vi "View one AI param scada restr.vi"(4 "AIParamTable":string="fa_1", 6 "OPC UA.Client refnum":T2, 7 "conninfo":T4={"host"="localhost", "port"="5432", "client_encoding"="WIN1251", "dbname"="system", "user"="postgres", "password"=""}, 8 "error in (no error)":errorcluster, 9 "AIParameters":string[](array[string]), 10 "AI_State":T3[](array[typedef]), 11 "AITable":dbl[](array[numeric]) format="%#.0f") -> (0 "error out":errorcluster)   [LabVIEW 2019]
uses:
  Ctl/AIParamColumns.ctl
  Inputs.lvlib
  <vilib>/OPCUA/controls/NodeId.ctl
  <vilib>/OPCUA/NI OPC UA Client.lvlib
  OPC/OPC addons.lvlib
  Ctl/View one AI param State.ctl
  <vilib>/Utility/miscctls.llb/LVRowAndColumnUnsignedTypeDef.ctl
  <vilib>/OPCUA/client/Multiple Write Variant.vi
  Ctl/Parameter State.ctl
  Database/ctl/Coninfo.ctl
  Database/PostgreSQL.lvlib
  <vilib>/OPCUA/controls/OPC UA Client Refnum.ctl
panel:
  in  "Tab Control":T1(tab)
  in  "input_register_min":dbl min=-32768.0 max=65535.0 step=1.0 format="%#.0f"
  in  "input_register_max":dbl min=-32768.0 max=65535.0 step=1.0 format="%#.0f"
  in  "input_pv_min":dbl format="%#.1f"
  in  "input_pv_max":dbl format="%#.1f"
  in  "instrument_gain":dbl min=-32768.0 max=65535.0 step=1.0 format="%#.0f"
  in  "instrument_offset":dbl min=-32768.0 max=65535.0 step=1.0 format="%#.0f"
  in  "sensor num":i32
  in  "instrument_min_offset":dbl min=-32768.0 max=65535.0 step=1.0 format="%#.0f"
  in  "time_const":dbl min=-32768.0 max=65535.0 step=1.0 format="%#.0f"
  in  "fcode_full":string="кгс/см2"
  out "AI_1":dbl format="%#.1f"
  in  "Param":i32(listbox) caption="Параметры"
  in  "d":dbl min=-32768.0 max=65535.0 step=1.0 format="%#.0f"
  in  "instrument_max_offset":dbl min=-32768.0 max=65535.0 step=1.0 format="%#.0f"
  out "units":string="кгс/см2"
  in  "instrument_range_max":dbl format="%#.1f"
  in  "process_range_max":dbl format="%#.1f"
  in  "process_high_acd":dbl format="%#.1f"
  in  "process_high_alr":dbl format="%#.1f"
  in  "process_low_alr":dbl format="%#.1f"
  in  "process_low_acd":dbl format="%#.1f"
  in  "process_range_min":dbl format="%#.1f"
  in  "instrument_range_min":dbl format="%#.1f"
  # "Настройка пределов"
  # "верхнийний предел датчика"
  # "верхний предел достоверных показаний"
  # "верхний аварийный предел"
  # "верхний предупредительный предел"
  # "нижний предупредительный предел"
  # "нижний аварийный предел"
  # "нижний предел достоверных показаний"
  # "нижний предел датчика"
  # "Y"
  # "значение сигнала максимум (Ymax)"
  # "значение сигнала минимум (Ymin)"
  # "X"
  # "входной регистр минимум (Xmin)"
  # "входной регистр максимум (Xmax)"
  # "Y"
  # "массштабирование"
  # "смещение"
  # "X"
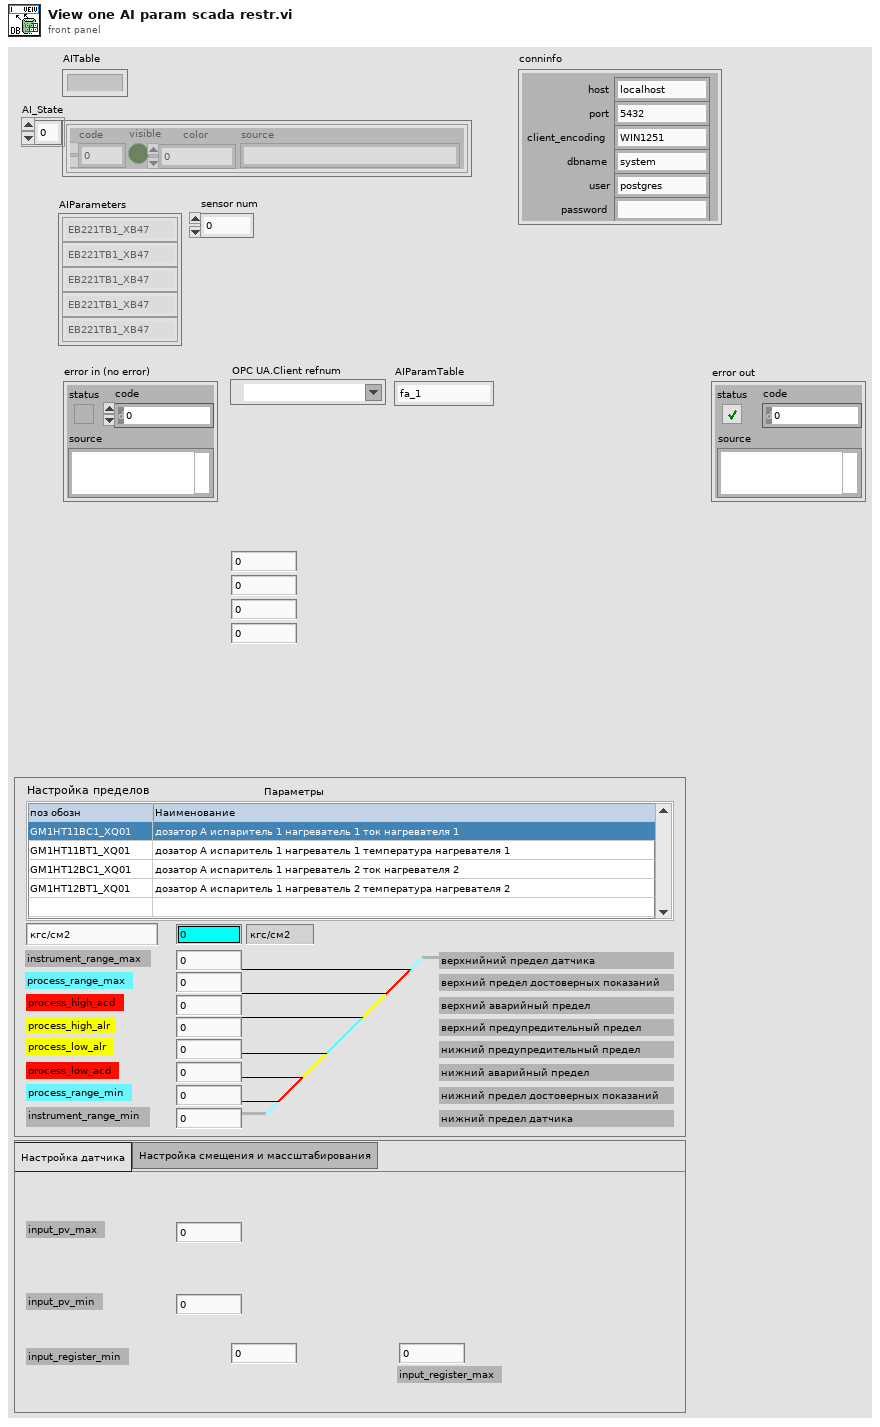
[diagram p1: front panel]
types:
  T1 = enum32{"Настройка датчика", "Настройка смещения и массштабирования"}
  T2 = typedef "OPC UA Client Refnum.ctl" = refnum<k21>
  T3 = typedef "Inputs.lvlib/Parameter State.ctl" = cluster{"code":i32, "visible":bool, "color":u32, "source":string}
  T4 = typedef "PostgreSQL.lvlib/Coninfo.ctl" = cluster{"host":string, "port":string, "client_encoding":string, "dbname":string, "user":string, "password":string}
  T5 = typedef "Inputs.lvlib/View one AI param State.ctl" = enum16{"init", "change sensor", "wait changes", "write parameters"}
  T6 = typedef "LVRowAndColumnUnsignedTypeDef.ctl" = cluster{"Row":u32, "Column":u32}
  T7 = typedef "NodeId.ctl" = string
  T8 = typedef "Inputs.lvlib/AIParamColumns.ctl" = enum16{"instrument_gain", "instrument_offset", "time_const", "instrument_min_offset", "instrument_range_min", "process_range_min", "process_low_acd", "process_low_alr", "process_high_alr", "process_high_acd", "process_range_max", "instrument_range_max", "instrument_max_offset", "d", "input_register_min", "input_register_max", "input_pv_min", "input_pv_max", "module_fcode_full", "control_channel_num", "ip_adress", "fcode", "fcodef", "fcode_full", "fname", "process_units"}
  T9 = typedef "Write Variant Request.ctl" = cluster{"node ID":T7, "value":variant, "timestamp (current time)":timestamp, "node status":T10}
  T10 = typedef "Write Status.ctl" = u32
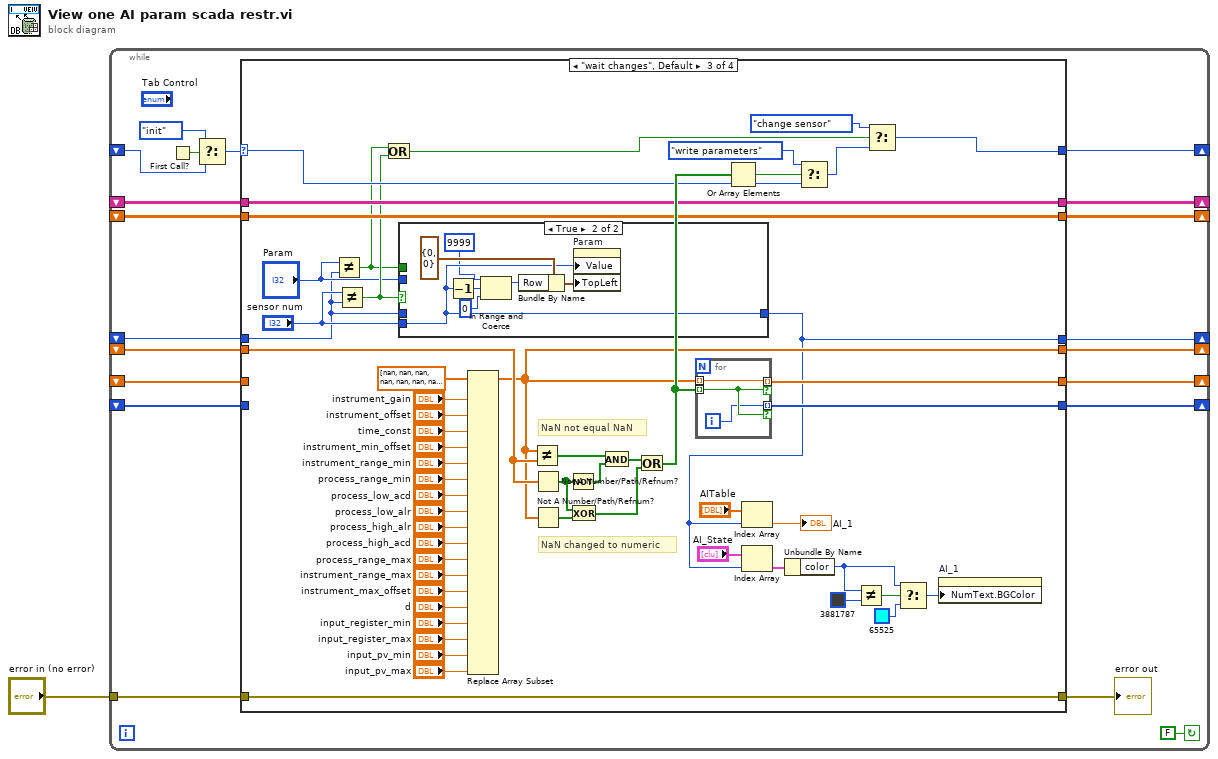
[diagram p0: block diagram]
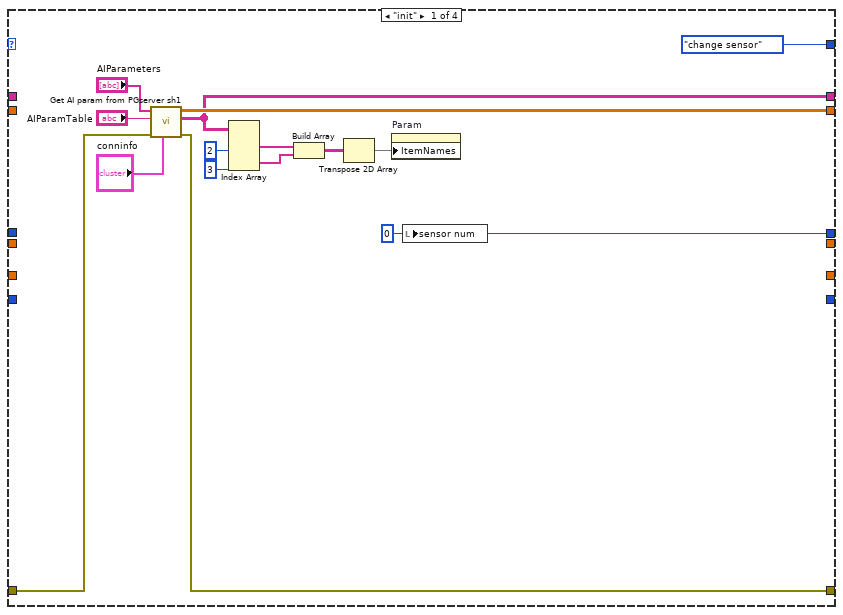
[diagram p2: hidden frame]
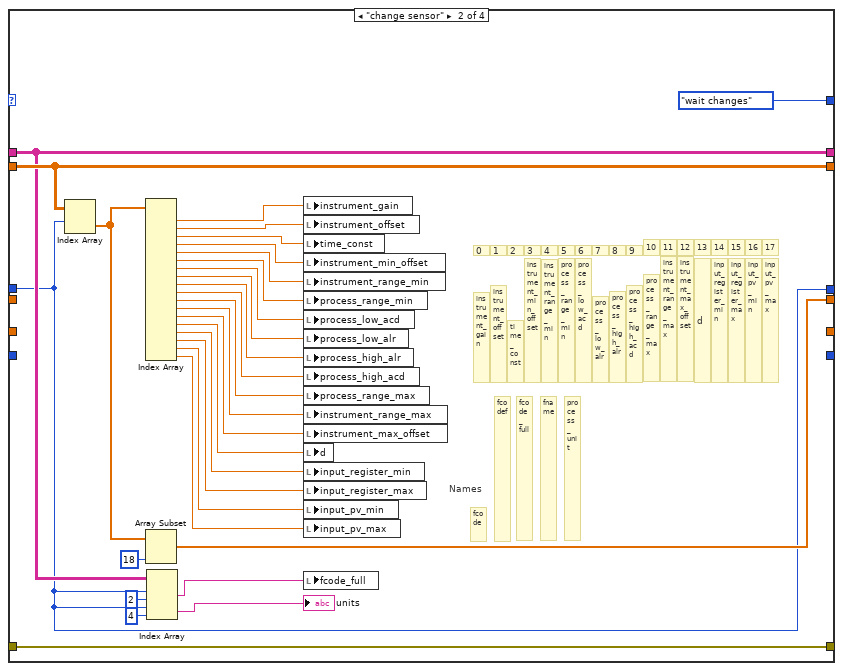
[diagram p3: hidden frame]
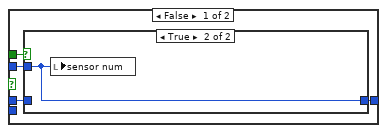
[diagram p4: hidden frame]
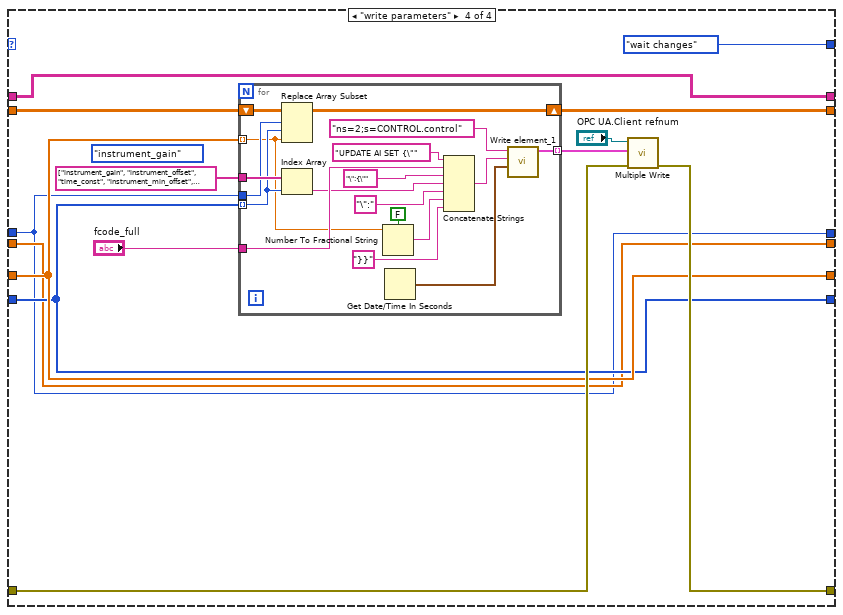
[diagram p6: hidden frame]
diagram:
  n1 = while {
    shift-right: [w19] -> _
    shift-left: _ -> [w17]
    shift-right: [w18] -> _
    shift-left: _ -> [w16]
    shift-right: [w15] -> _
    shift-left: _ -> [w14]
    tunnel: "error in (no error)" -> [w13]
    shift-right: [w12] -> _
    shift-left: _ -> [w4]
    shift-right: [w11] -> _
    shift-left: _ -> [w9]
    shift-right: [w10] -> _
    shift-left: _ -> [w8]
    shift-right: [w7] -> _
    shift-left: _ -> [w6]
    stop <- FALSE ("Boolean") continue-if-true
    n2 = First Call?() -> (First Call?: T/F=w5:bool)
    n3 = Select(t=View_one_AI_param_State."init", s=w5, f=w4) -> (s? t:f=w2:T5)
    n4 = case shown="\"wait changes\", Default" w2 {
      selector: w2 -> [_ _ w82 _]
      tunnel: w6 -> [_ w37 w73 w138]
      tunnel: w16 -> [_ w48 w93 w148]
      tunnel: w17 -> [_ w49 w88 w150]
      tunnel: [w29 w39 w85 w151] -> w21
      tunnel: [_ w47 w99 w139] -> w15
      tunnel: w14 -> [_ _ w102 w139]
      tunnel: [w31 w49 w88 w149] -> w19
      tunnel: [w28 w48 w93 w148] -> w18
      tunnel: w13 -> [w30 w39 w85 w147]
      tunnel: [View_one_AI_param_State."change sensor" View_one_AI_param_State."wait changes" w81 View_one_AI_param_State."wait changes"] -> w12
      tunnel: [_ _ w87 w141] -> w11
      tunnel: [_ _ w86 w140] -> w10
      tunnel: w9 -> [_ _ _ w141]
      tunnel: w8 -> [_ _ _ w140]
      tunnel: [w22 w37 w72 w138] -> w7
      frame "init" {
        w22 = 0 ("sensor num")
        n5 = call "Get AI param from PGserver sh1.vi"("conninfo"="conninfo", "error in (no error)"=w30, "AIParamTable"="AIParamTable", "AIParameters"="AIParameters") -> ("error out"=w29:errorcluster, "Names table"=w28:string[][], "Parameters table"=w31:dbl[][])  [unwired: 5 in]
        n6 = Index Array(array=w28, index (col) #1=2 ("index (row)"), index (col) #2=3 ("index (row)")) -> (element #1=w26:string[], element #2=w25:string[])  [unwired: 2 in]
        n7 = Build Array(w26, w25) -> (w24:string[][])
        n8 = Transpose 2D Array(2D array=w24) -> (transposed array=w23:string[][])
        n9 = property on="Param" class="MCListbox (strict)"("ItemNames"=w23) -> ()  [unwired: 2 in, 2 out]
        n10 = local write "sensor num"(w22) -> ()
      }
      frame "change sensor" {
        # "fcodef"
        # "process_unit"
        # "fname"
        # "fcode_full"
        # "fcode"
        # "Names"
        # "input_pv_max"
        # "input_pv_min"
        # "input_register_max"
        # "input_register_min"
        # "d"
        # "instrument_max_offset"
        # "instrument_range_max"
        # "process_range_max"
        # "process_high_acd"
        # "process_high_alr"
        # "process_low_alr"
        # "process_low_acd"
        # "process_range_min"
        # "instrument_range_min"
        # "instrument_min_offset"
        # "time_const"
        # "instrument_gain"
        # "instrument_offset"
        # "17"
        # "16"
        # "15"
        # "14"
        # "13"
        # "12"
        # "11"
        # "10"
        # "9"
        # "8"
        # "7"
        # "6"
        # "5"
        # "4"
        # "3"
        # "2"
        # "0"
        # "1"
        n11 = Index Array(array=w49, index (row)=w37) -> (element=w51:dbl[])  [unwired: 1 in]
        n12 = Index Array(array=w51) -> (element #1=w41:dbl, element #2=w42:dbl, element #3=w43:dbl, element #4=w44:dbl, element #5=w65:dbl, element #6=w64:dbl, element #7=w63:dbl, element #8=w62:dbl, element #9=w61:dbl, element #10=w60:dbl, element #11=w59:dbl, element #12=w58:dbl, element #13=w53:dbl, element #14=w52:dbl, element #15=w57:dbl, element #16=w56:dbl, element #17=w55:dbl, element #18=w54:dbl)  [unwired: 18 in]
        n13 = Array Subset(array=w51, length=18) -> (w47:dbl[])  [unwired: 1 in]
        n14 = Index Array(array=w48, index (row) #1=w37, index (col) #1=2 ("length"), index (row) #2=w37, index (col) #2=4 ("length")) -> (element #1=w40:string, element #2=→"units":string)
        n15 = local write "instrument_gain"(w41) -> ()
        n16 = local write "instrument_offset"(w42) -> ()
        n17 = local write "time_const"(w43) -> ()
        n18 = local write "instrument_min_offset"(w44) -> ()
        n19 = local write "instrument_range_min"(w65) -> ()
        n20 = local write "process_range_min"(w64) -> ()
        n21 = local write "process_low_acd"(w63) -> ()
        n22 = local write "process_low_alr"(w62) -> ()
        n23 = local write "process_high_alr"(w61) -> ()
        n24 = local write "process_high_acd"(w60) -> ()
        n25 = local write "process_range_max"(w59) -> ()
        n26 = local write "instrument_range_max"(w58) -> ()
        n27 = local write "instrument_max_offset"(w53) -> ()
        n28 = local write "d"(w52) -> ()
        n29 = local write "input_register_min"(w57) -> ()
        n30 = local write "input_register_max"(w56) -> ()
        n31 = local write "input_pv_min"(w55) -> ()
        n32 = local write "input_pv_max"(w54) -> ()
        n33 = local write "fcode_full"(w40) -> ()
      }
      frame "wait changes", Default {
        # "NaN changed to numeric"
        # "NaN not equal NaN"
        n34 = Not Equal?(x="Param", y=w73) -> (x != y?=w76:bool)
        n35 = Not Equal?(x="sensor num", y=w73) -> (x != y?=w78:bool)
        n36 = Or(x=w76, y=w78) -> (x .or. y?=w77:bool)
        n37 = case shown="True" w78 {
          tunnel: "sensor num" -> [_ w130]
          tunnel: w76 -> [w125 _]
          tunnel: [w123 w130] -> w72
          tunnel: "Param" -> [w124 _]
          tunnel: w73 -> [w122 _]
          frame False {
            n38 = case shown="True" w125 {
              tunnel: w124 -> [_ w127]
              tunnel: [w126 w127] -> w123
              tunnel: w122 -> [w126 _]
              frame False {
              }
              frame True {
                n39 = local write "sensor num"(w127) -> ()
              }
            }
          }
          frame True {
            n40 = Decrement(x=w130) -> (x-1=w131:i32)
            n41 = In Range and Coerce(upper limit=9999, x=w131, lower limit=0) -> (coerced(x)=w132:i32)  [unwired: 1 out]
            n42 = Bundle By Name(cluster=T6 {"Row"=0, "Column"=0} ("Top Left Visible Cell"), "Row"=w132) -> (w133:T6)
            n43 = property on="Param" class="MCListbox (strict)"("Value"=w130, "TopLeft"=w133) -> ()  [unwired: 2 in, 2 out]
          }
        }
        n44 = Replace Array Subset(array=dbl[] [nan, nan, nan, nan, nan, nan, nan, nan, nan, nan, nan, nan, nan, nan, nan, nan, nan, nan] ("Parameters table"), new element #1="instrument_gain", new element #2="instrument_offset", new element #3="time_const", new element #4="instrument_min_offset", new element #5="instrument_range_min", new element #6="process_range_min", new element #7="process_low_acd", new element #8="process_low_alr", new element #9="process_high_alr", new element #10="process_high_acd", new element #11="process_range_max", new element #12="instrument_range_max", new element #13="instrument_max_offset", new element #14="d", new element #15="input_register_min", new element #16="input_register_max", new element #17="input_pv_min", new element #18="input_pv_max") -> (w99:dbl[])  [unwired: 18 in]
        n45 = Not Equal?(x=w99, y=w102) -> (x != y?=w100:bool[])
        n46 = Not A Number/Path/Refnum?(number/path/refnum=w102) -> (NaN/Path/Refnum?=w95:bool[])
        n47 = Not A Number/Path/Refnum?(number/path/refnum=w99) -> (NaN/Path/Refnum?=w94:bool[])
        n48 = Not(x=w95) -> (.not. x?=w96:bool[])
        n49 = Exclusive Or(1:w94, 2:w95) -> (0:w98:bool[])
        n50 = And(x=w100, y=w96) -> (x .and. y?=w97:bool[])
        n51 = Or(x=w97, y=w98) -> (x .or. y?=w101:bool[])
        n52 = for {
          tunnel: w99 -> [w137] mode=indexing
          tunnel: w101 -> [w136] mode=indexing
          tunnel: [w137] -> w87 mode=indexing if=w136
          tunnel: [w135] -> w86 mode=indexing if=w136
          i -> [w135]
        }
        n53 = Or Array Elements(Boolean array=w101) -> (logical OR=w83:bool)
        n54 = Index Array(array="AITable", index=w72) -> (element=→"AI_1":dbl)
        n55 = Index Array(array="AI_State", index=w72) -> (element=w103:T3)
        n56 = Unbundle By Name(w103) -> ("color"=w69:u32)
        n57 = Select(t=View_one_AI_param_State."write parameters", s=w83, f=w82) -> (s? t:f=w80:T5)
        n58 = Not Equal?(x=w69, y=u32 3881787 ("color")) -> (x != y?=w70:bool)
        n59 = Select(t=View_one_AI_param_State."change sensor", s=w77, f=w80) -> (s? t:f=w81:T5)
        n60 = Select(t=w69, s=w70, f=u32 65525 ("color")) -> (s? t:f=w68:u32)
        n61 = property on="AI_1" class="DigNum (strict)"("NumText.BGColor"=w68) -> ()  [unwired: 2 in, 2 out]
      }
      frame "write parameters" {
        (unwired) AIParamColumns."instrument_gain" ("AIParamColumns")
        n62 = for {
          tunnel: w138 -> [w166]
          tunnel: string[] ["instrument_gain", "instrument_offset", "time_const", "instrument_min_offset", "instrument_range_min", "process_range_min", "process_low_acd", "process_low_alr", "process_high_alr", "process_high_acd", "process_range_max", "instrument_range_max", "instrument_max_offset", "d", "input_register_min", "input_register_max", "input_pv_min", "input_pv_max", "fcode", "fcodef", "fcode_full", "fname", "process_units"] ("AIParamColumns") -> [w169]
          tunnel: w140 -> [w163] mode=indexing
          tunnel: w141 -> [w154] mode=indexing
          shift-right: [w167] -> w149
          shift-left: w150 -> [w168]
          tunnel: "fcode_full" -> [w156]
          tunnel: [w152] -> w144 mode=indexing
          n63 = Replace Array Subset(array=w168, new element=w154, index (row)=w166, index (col)=w163) -> (w167:dbl[][])
          n64 = Index Array(array=w169, index=w163) -> (element=w155:string)
          n65 = Number To Fractional String(use system decimal point (T)=FALSE, number=w154) -> (F-format string=w162:string)  [unwired: 2 in]
          n66 = Get Date/Time In Seconds() -> (seconds since 1Jan1904=w164:timestamp)
          n67 = Concatenate Strings("UPDATE AI SET {\"" ("string"), w156, "\":{\"" ("string"), w155, "\":" ("string"), w162, "}}" ("string")) -> (w153:string)
          n68 = call "Write element_1.vi"("seconds since 1Jan1904"=w164, "Variant"=w153, "node ID"=T7 "ns=2;s=CONTROL.control") -> ("request out"=w152:T9)  [unwired: 8 in]
        }
        n69 = call-poly <vilib>:"Multiple Write.vi"("error in (no error)"=w147, "requests"=w144, "OPC UA client refnum in"="OPC UA.Client refnum") -> ("error out"=w151:errorcluster)  [unwired: 5 in, 3 out]
      }
    }
    "error out" <- w21
  }
